vi "Event Wait.vi"(8 "error in (no error)":errorcluster, 11 "Event DVR in":refnum<data-value>) -> (0 "error out":errorcluster, 3 "Event DVR out":refnum<data-value>)   [LabVIEW 2010, in "MDSplus.lvlib"]
doc: "Return data received last."
uses:
  <vilib>/MDSplus/Library/MDSplus.lvlib
  <vilib>/MDSplus/Classes/Event_Class/Event.lvclass
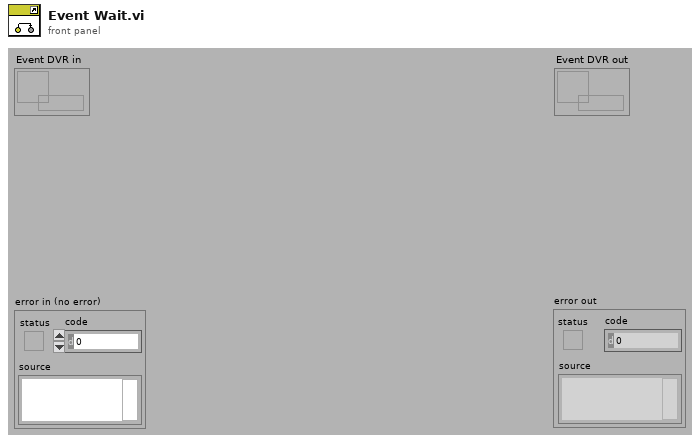
[diagram p1: front panel]
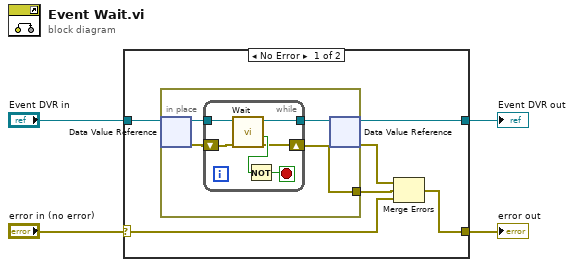
[diagram p0: block diagram]
diagram:
  n1 = case shown="No Error" "error in (no error)" {
    selector: "error in (no error)" -> [w9 w22]
    tunnel: "Event DVR in" -> [w10 w21]
    tunnel: [w6 w22] -> w4
    tunnel: [w7 w21] -> w1
    frame No Error {
      n2 = in-place {
        in-place-border: [w11] -> w5
        n3 = in-place-dvr #1(w10) -> (w14:refnum<class "Event.lvclass">, w13:errorcluster)
        n4 = while {
          tunnel: w14 -> [w16]
          tunnel: [w15] -> w12
          shift-right: [w17] -> w11
          shift-left: w13 -> [w20]
          stop <- w18 stop-if-true
          n5 = call-dynamic "Wait.vi"("error in (no error)"=w20, "Event in"=w16) -> ("error out"=w17:errorcluster, "Timeout Occurred"=w19:bool, "Event out"=w15:refnum<class "Event.lvclass">)  [unwired: 7 in]
          n6 = Not(x=w19) -> (.not. x?=w18:bool)
        }
        n7 = in-place-dvr #1(w12) -> (w7:refnum<data-value>, w8:errorcluster)
      }
      n8 = Merge Errors(w8, w5, w9) -> (w6:errorcluster)
    }
    frame Error {
    }
  }
  "error out" <- w4
  "Event DVR out" <- w1
